vi "ReadWait.vi"(8 "error in (no error)":errorcluster, 9 "Value":bool=TRUE, 10 "Read":i32, 11 "I-O in":refnum<class "I-O.lvclass">) -> (0 "error out":errorcluster, 3 "I-O out":refnum<class "I-O.lvclass">)   [LabVIEW 2016, in "I-O.lvclass"]
uses:
  I-O.lvclass
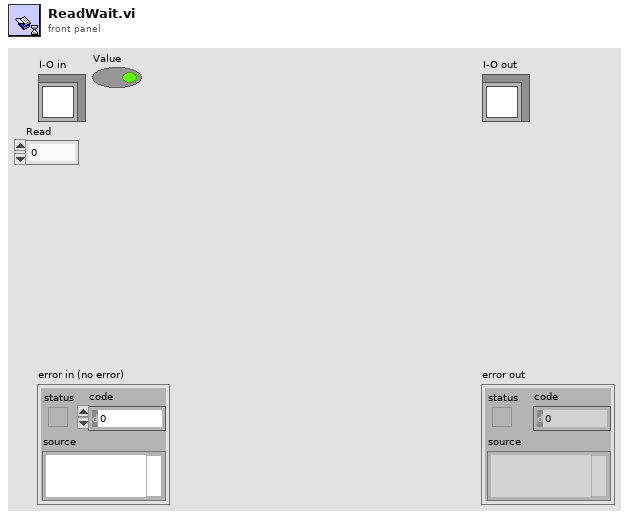
[diagram p1: front panel]
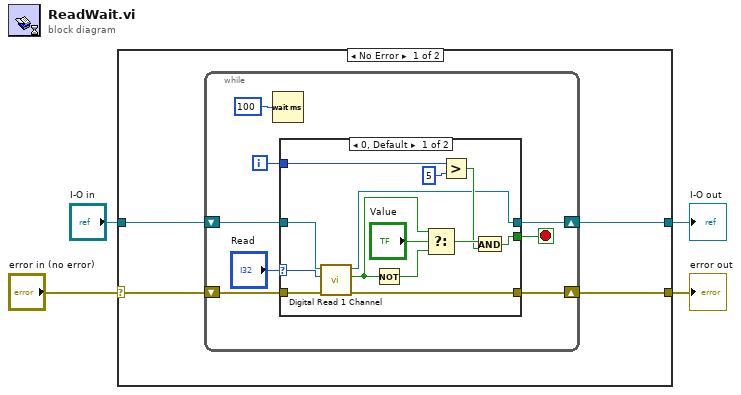
[diagram p0: block diagram]
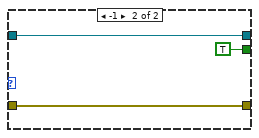
[diagram p2: hidden frame]
diagram:
  n1 = case shown="No Error" "error in (no error)" {
    selector: "error in (no error)" -> [w8 w34]
    tunnel: [w7 w34] -> w3
    tunnel: [w5 w33] -> w1
    tunnel: "I-O in" -> [w6 w33]
    frame No Error {
      n2 = while {
        shift-right: [w12] -> w5
        shift-left: w6 -> [w13]
        shift-right: [w10] -> w7
        shift-left: w8 -> [w11]
        i -> [w15]
        stop <- w14 stop-if-true
        n3 = Wait (ms)(milliseconds to wait=u32 100) -> ()  [unwired: 1 out]
        n4 = case shown="0, Default" "Read" {
          selector: "Read" -> [w18 _]
          tunnel: w15 -> [w28 _]
          tunnel: [w24 TRUE] -> w14
          tunnel: w13 -> [w23 w32]
          tunnel: [w21 w32] -> w12
          tunnel: w11 -> [w20 w30]
          tunnel: [w19 w30] -> w10
          frame 0, Default {
            n5 = call-dynamic "Digital Read 1 Channel.vi"("error in (no error)"=w20, "Read"=w18, "I-O in"=w23) -> ("error out"=w19:errorcluster, "Value"=w22:bool, "I-O out"=w21:refnum<class "I-O.lvclass">)  [unwired: 6 in]
            n6 = Not(x=w22) -> (.not. x?=w29:bool)
            n7 = Select(t=w22, s="Value", f=w29) -> (s? t:f=w26:bool)
            n8 = Greater?(x=w28, y=5) -> (0:w25:bool)
            n9 = And(x=w26, y=w25) -> (x .and. y?=w24:bool)
          }
          frame -1 {
          }
        }
      }
    }
    frame Error {
    }
  }
  "error out" <- w3
  "I-O out" <- w1
